vi "$FKXX.vi"(11 "反馈信息":string) -> (3 "接收信息":T1 {"信息内容"."反馈标志" items=["成功", "失败", "信号未锁定", "电量不足", "发射频度未到", "加解密错误", "CRC错误"]})   [LabVIEW 2016, in "环境动力监测库.lvlib" / "NMEA.lvlib"]
uses:
  NMEA.lvlib
panel:
  # "Bus Hound 6.01 capture on Windows Vista Service Pack 1 (x64). Complements of www.perisoft.net\n\n  Device - Device ID (followed by the endpoint for USB devices)\n            (6) 通信端口 (COM3)\n            (13) Prolific USB-to-Serial Comm Port (COM9)\n            (14) Unknown Device\n            (15) Unknown Device\n            (18) Microsoft Serial BallPoint\n  Phase  - Phase Type\n            IN    Data in transfer           \n            OUT   Data out transfer          \n  Data   - Hex dump of the data transferred\n  Descr  - Description of the phase\n  Cmd... - Position in the captured data\n\n\nDevice  Phase  Data                      Description       Cmd.Phase.Ofs(rep)\n------  -----  ------------------------  ----------------  ------------------\n   6    IN     24 46 4b 58  58 00 10 0e  $FKXX...                79.1.0        \n               c6 75 04 1b  00 00        .u....                  79.1.8        \n   6    IN     00 9b                     ..                      80.1.0"
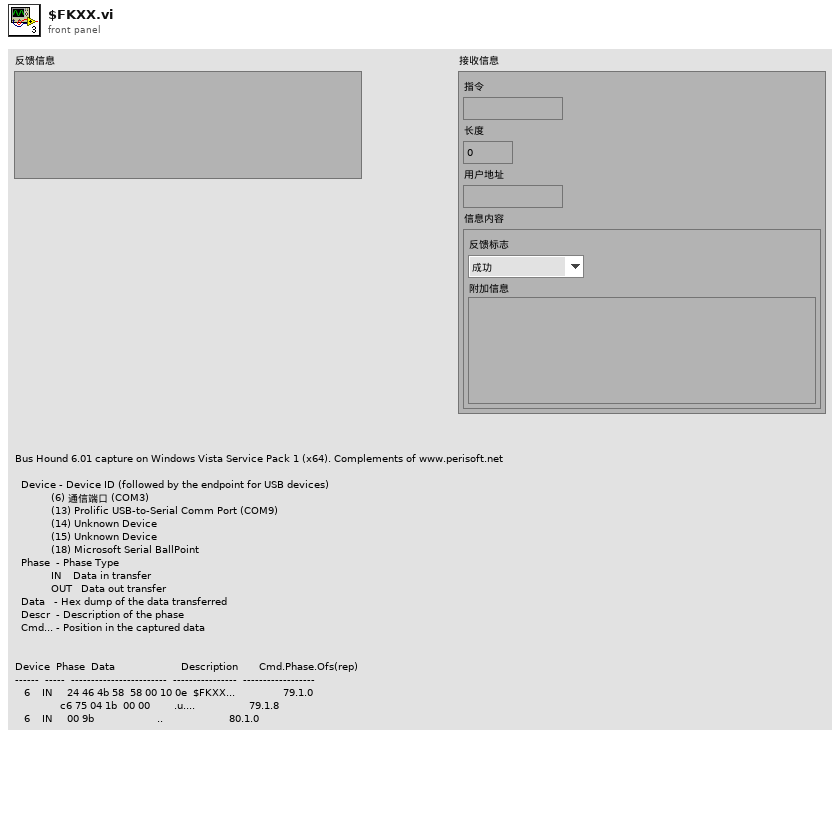
[diagram p1: front panel]
types:
  T1 = cluster{"指令":string, "长度":u16, "用户地址":string, "信息内容":cluster{"反馈标志":u16, "附加信息":string}}
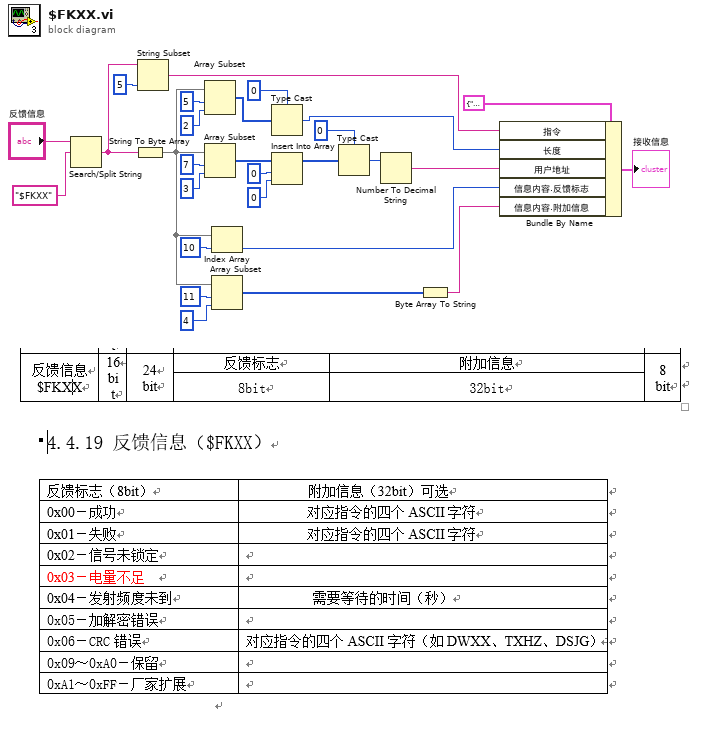
[diagram p0: block diagram]
diagram:
  n1 = Search/Split String(string="反馈信息", search string/char (-)="$FKXX" ("搜索字符串/字符(-)")) -> (match + rest of string=w21:string)  [unwired: 1 in, 2 out]
  n2 = String To Byte Array(string=w21) -> (unsigned byte array=w4:u8[])
  n3 = String Subset(string=w21, length (rest)=5 ("长度（剩余）")) -> (substring=w18:string)  [unwired: 1 in]
  n4 = Array Subset(array=w4, index=5 ("索引"), length=2 ("长度")) -> (w15:u8[])
  n5 = Array Subset(array=w4, index=7 ("索引"), length=3 ("长度")) -> (w10:u8[])
  n6 = Index Array(array=w4, index=10 ("索引")) -> (element=w2:u8)
  n7 = Array Subset(array=w4, index=11 ("索引"), length=4 ("长度")) -> (w25:u8[])
  n8 = Type Cast(type=u16 0 ("长度"), x=w15) -> (*(type *) &x=w13:u16)
  n9 = Insert Into Array(array=w10, index=0 ("索引"), new element=u8 0 ("新元素/子数组")) -> (w7:u8[])
  n10 = Type Cast(type=u32 0 ("长度"), x=w7) -> (*(type *) &x=w8:u32)
  n11 = Number To Decimal String(number=w8) -> (decimal integer string=w3:string)  [unwired: 1 in]
  n12 = Byte Array To String(unsigned byte array=w25) -> (string=w1:string)
  n13 = Bundle By Name(cluster=T1 {"指令"="", "长度"=0, "用户地址"="", "信息内容"={"反馈标志"=0, "附加信息"=""}} ("接收信息"), "指令"=w18, "长度"=w13, "用户地址"=w3, "信息内容.反馈标志"=w2, "信息内容.附加信息"=w1) -> (→"接收信息":T1)
